vi "envoi mail valves expediées.vi"(4 "tab histo filtré\n par n° cmde":string[][](array[string]), 7 "DIVISION":enum16{"FLATPROP", "MEDIC"}(ring), 8 "error in (no error)":errorcluster caption="entrée d'erreur (pas d'erreur)", 10 "DATA cmde":T1, 11 "chaine valves":string="12-216C-04521 EQIFIL 417mA 14.4ohm\t112105740008030109\t18.04.2008 15:35\tMQI\t12345/06-03.03.03\t2\t30\r\n12-216C-04521 EQIFIL 417mA 14.4ohm\t112105740008030108\t18.04.2008 15:35\tMQI\t12345/06-03.03.03\t2\t30\r\n12-216C-04521 EQIFIL 417mA 14.4ohm\t112105740008030107\t18.04.2008 15:35\tMQI\t12345/06-03.03.03\t2\t30\r\n12-216C-04521 EQIFIL 417mA 14.4ohm\t112105740008030106\t18.04.2008 15:35\tMQI\t12345/06-03.03.03\t2\t30\r\n12-216C-04521 EQIFIL 417mA 14.4ohm\t112105740008030105\t18.04.2008 15:35\tMQI\t12345/06-03.03.03\t2\t30\r\n12-216C-04521 EQIFIL 417mA 14.4ohm\t112105740008030104\t18.04.2008 15:35\tMQI\t12345/06-03.03.03\t1\t30\r\n12-216C-04521 EQIFIL 417mA 14.4ohm\t112105740008030103\t18.04.2008 15:34\tMQI\t12345/06-03.03.03\t1\t30\r\n12-216C-04521 EQIFIL 417mA 14.4ohm\t112105740008030102\t18.04.2008 15:34\tMQI\t12345/06-03.03.03\t1\t30\r\n12-216C-04521 EQIFIL 417mA 14.4ohm\t112105740008030101\t18.04.2008 15:34\tMQI\t12345/06-03.03.03\t1\t30\r\n12-216C-04521 EQIFIL 417mA 14.4ohm\t112105740008030100\t18.04.2008 15:34\tMQI\t12345/06-03.03.03\t1\t30\r\n12-216C-04521 EQIFIL 417mA 14.4ohm\t112105740008020106\t18.04.2008 15:34\tMQI\t12345/06-03.03.03\t1\t30\r\n12-216C-04521 EQIFIL 417mA 14.4ohm\t112105740008020105\t18.04.2008 15:34\tMQI\t12345/06-03.03.03\t1\t30\r\n12-216C-04521 EQIFIL 417mA 14.4ohm\t112105740008020104\t18.04.2008 15:34\tMQI\t12345/06-03.03.03\t1\t30\r\n12-216C-04521 EQIFIL 417mA 14.4ohm\t112105740008020103\t18.04.2008 15:34\tMQI\t12345/06-03.03.03\t1\t30\r\n12-216C-04521 EQIFIL 417mA 14.4ohm\t112105740008020102\t18.04.2008 15:34\tMQI\t12345/06-03.03.03\t1\t30\r\n12-216C-04521 EQIFIL 417mA 14.4ohm\t112105740008020101\t18.04.2008 15:34\tMQI\t12345/06-03.03.03\t1\t30\r\n12-216C-04521 EQIFIL 417mA 14.4ohm\t112105740008020100\t18.04.2008 15:34\tMQI\t12345/06-03.03.03\t1\t30\r\n12-216C-04521 EQIFIL 417mA 14.4ohm\t112105740008010112\t18.04.2008 15:34\tMQI\t12345/06-03.03.03\t1\t30\r\n12-216C-04521 EQIFIL 417mA 14.4ohm\t112105740008010111\t18.04.2008 15:34\tMQI\t12345/06-03.03.03\t1\t30\r\n12-216C-04521 EQIFIL 417mA 14.4ohm\t112105740008010110\t18.04.2008 15:34\tMQI\t12345/06-03.03.03\t1\t30\r\n12-216C-04521 EQIFIL 417mA 14.4ohm\t112105740008010109\t18.04.2008 15:34\tMQI\t12345/06-03.03.03\t1\t30\r\n12-216C-04521 EQIFIL 417mA 14.4ohm\t112105740008010108\t18.04.2008 15:34\tMQI\t12345/06-03.03.03\t1\t30\r\n12-216C-04521 EQIFIL 417mA 14.4ohm\t112105740008010107\t18.04.2008 15:34\tMQI\t12345/06-03.03.03\t1\t30\r\n12-216C-04521 EQIFIL 417mA 14.4ohm\t112105740008010106\t18.04.2008 15:34\tMQI\t12345/06-03.03.03\t1\t30\r\n12-216C-04521 EQIFIL 417mA 14.4ohm\t112105740008010105\t18.04.2008 15:34\tMQI\t12345/06-03.03.03\t1\t30\r\n12-216C-04521 EQIFIL 417mA 14.4ohm\t112105740008010104\t18.04.2008 15:34\tMQI\t12345/06-03.03.03\t1\t30\r\n12-216C-04521 EQIFIL 417mA 14.4ohm\t112105740008010103\t18.04.2008 15:33\tMQI\t12345/06-03.03.03\t1\t30\r\n12-216C-04521 EQIFIL 417mA 14.4ohm\t112105740008010102\t18.04.2008 15:33\tMQI\t12345/06-03.03.03\t1\t30\r\n12-216C-04521 EQIFIL 417mA 14.4ohm\t112105740008010101\t18.04.2008 15:33\tMQI\t12345/06-03.03.03\t1\t30\r\n12-216C-04521 EQIFIL 417mA 14.4ohm\t112105740008010100\t18.04.2008 15:33\tMQI\t12345/06-03.03.03\t1\t30\r\n") -> (0 "error out":errorcluster caption="sortie d'erreur")   [LabVIEW 2020]
doc: "Envoi un mail avec la liste des valves emballées en pièce jointe si spécifié dans le fichier XML PP de la valve (FlatProp) ou correspondance produit code barre.txt (autres valves)"
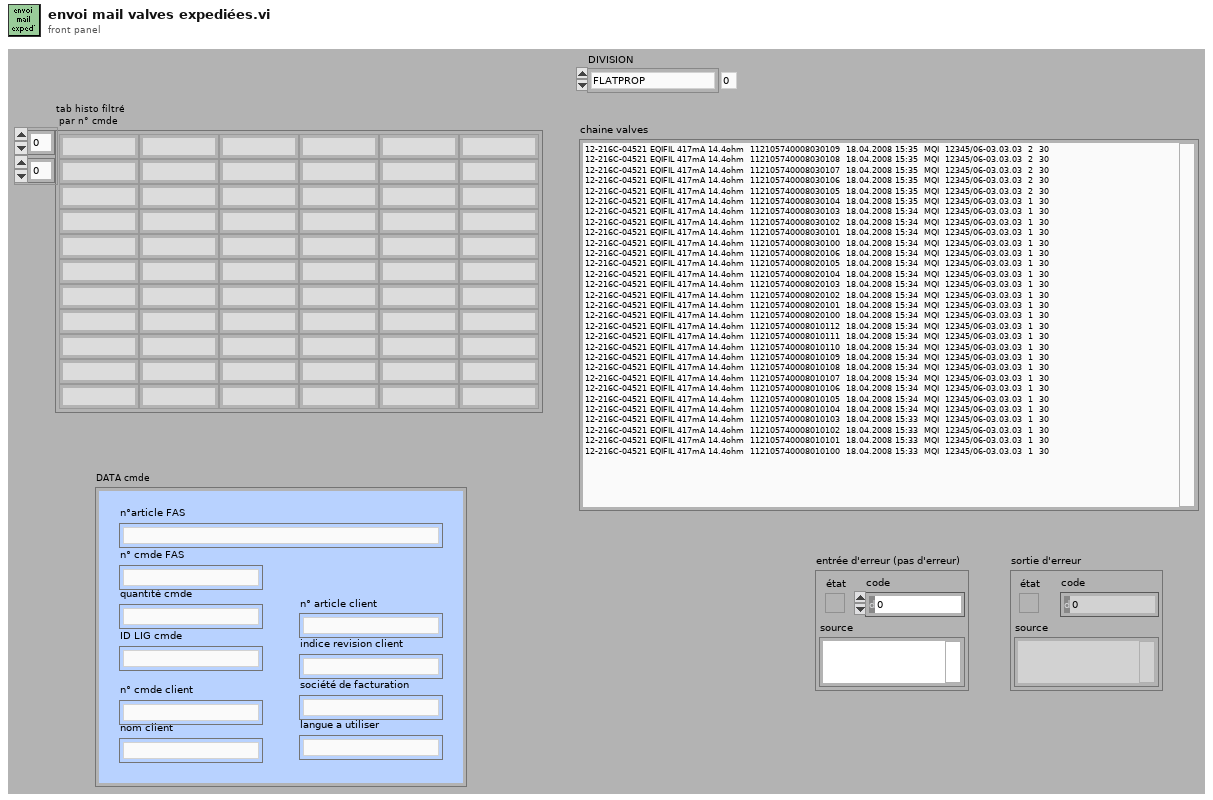
[diagram p1: front panel]
types:
  T1 = typedef "DATA commande.ctl" = cluster{"n°article FAS":string, "n° cmde FAS":string, "quantité cmde":string, "ID LIG cmde":string, "n° cmde client":string, "nom client":string, "n° article client":string, "indice revision client":string, "société de facturation":string, "langue a utiliser":string}
  T2 = enum16{"open", "replace", "create", "open or create", "replace or create", "replace or create with confirmation"}
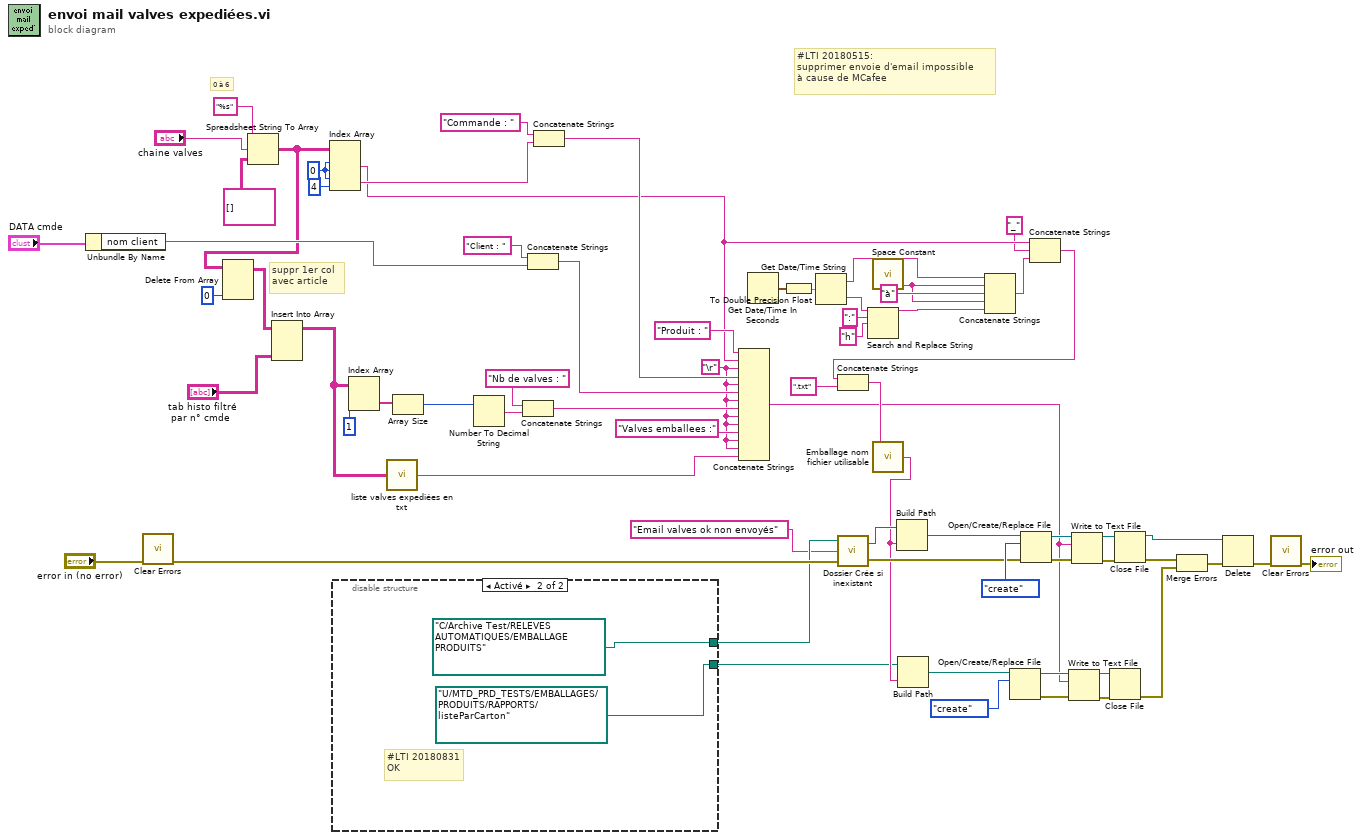
[diagram p0: block diagram]
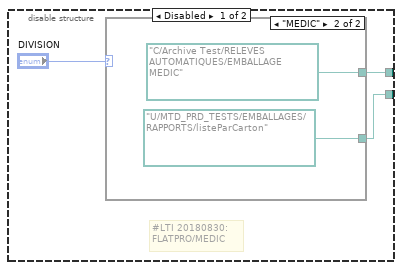
[diagram p2: hidden frame]
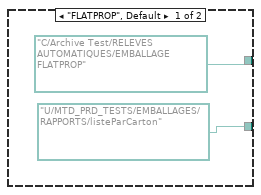
[diagram p3: hidden frame]
diagram:
  w52 = 0 ("indice désactivé (col)")
  w38 = "\r"
  # "#LTI 20180515:\nsupprimer envoie d'email impossible \nà cause de MCafee"
  # "suppr 1er col \navec article"
  # "0 à 6"
  n1 = Unbundle By Name("DATA cmde") -> ("nom client"=w65:string)
  n2 = call <vilib>:"Clear Errors.vi"("error in (no error)"="error in (no error)") -> ("error out"=w67:errorcluster)  [unwired: 5 in, 1 out]
  n3 = Spreadsheet String To Array(format string="%s" ("chaîne de format"), spreadsheet string="chaine valves", array type (2D Dbl)=string[][] [] ("type de tableau (2D de dbl)")) -> (array=w19:string[][])  [unwired: 1 in]
  n4 = Delete From Array(array=w19, index (col)=0 ("indice désactivé (col)")) -> (array with subset deleted=w17:string[][])  [unwired: 2 in, 1 out]
  n5 = Insert Into Array(array=w17, new element="tab histo filtré\n par n° cmde") -> (w14:string[][])  [unwired: 2 in]
  n6 = Index Array(array=w19, index (row) #1=w52, index (col) #1=w52, index (row) #2=w52, index (col) #2=4 ("indice désactivé (col)")) -> (element #1=w36:string, element #2=w50:string)
  n7 = disable-structure shown="Activé" {
    disable-tunnel: [w72 path "C:/Archive Test/RELEVES AUTOMATIQUES/EMBALLAGE PRODUITS" ("chemin local RELEVES AUTOM\\EMBALL_...")] -> w34
    disable-tunnel: [w70 path "U:/MTD_PRD_TESTS/EMBALLAGES/PRODUITS/RAPPORTS/listeParCarton" ("chemin local RELEVES AUTOM\\EMBALL_...")] -> w11
    frame Disabled {
      # "#LTI 20180830:\nFLATPRO/MEDIC"
      n8 = case shown="\"MEDIC\"" "DIVISION" {
        tunnel: [path "C:/Archive Test/RELEVES AUTOMATIQUES/EMBALLAGE FLATPROP" ("chemin local RELEVES AUTOM\\EMBALL_...") path "C:/Archive Test/RELEVES AUTOMATIQUES/EMBALLAGE MEDIC" ("chemin local RELEVES AUTOM\\EMBALL_...")] -> w72
        tunnel: [path "U:/MTD_PRD_TESTS/EMBALLAGES/RAPPORTS/listeParCarton" ("chemin local RELEVES AUTOM\\EMBALL_...") path "U:/MTD_PRD_TESTS/EMBALLAGES/RAPPORTS/listeParCarton" ("chemin local RELEVES AUTOM\\EMBALL_...")] -> w70
        frame "FLATPROP", Default {
        }
        frame "MEDIC" {
        }
      }
    }
    frame Enabled {
      # "#LTI 20180831\nOK"
    }
  }
  n9 = Index Array(array=w14, index (col)=1 ("indice désactivé (col)")) -> (element=w47:string[])  [unwired: 1 in]
  n10 = call "liste valves expediées en txt.vi"("Tab valves"=w14) -> ("liste valves"=w39:string)
  n11 = Array Size(array=w47) -> (size(s)=w16:i32)
  n12 = Number To Decimal String(number=w16) -> (decimal integer string=w45:string)  [unwired: 1 in]
  n13 = Concatenate Strings("Nb de valves : " ("expression régulière"), w45) -> (w62:string)
  n14 = Concatenate Strings("Client : " ("expression régulière"), w65) -> (w40:string)
  n15 = Concatenate Strings("Commande : " ("expression régulière"), w50) -> (w63:string)
  n16 = Concatenate Strings("Produit : " ("expression régulière"), w36, w38, w63, w38, w40, w38, w62, w38, w38, "Valves emballees :" ("chaîne"), w38, w38, w39) -> (w2:string)
  n17 = Get Date/Time In Seconds() -> (seconds since 1Jan1904=w28:timestamp)
  n18 = To Double Precision Float(number=w28) -> (double precision float=w29:dbl)
  n19 = Get Date/Time String(seconds (now)=w29) -> (date string=w22:string, time string=w25:string)  [unwired: 2 in]
  n20 = call "Dossier Crée si inexistant.vi"("error in"=w67, "nom sous dossier"="Email valves ok non envoyés", "chemin du dossier IN"=w34) -> ("error out"=w33:errorcluster, "chemin sous dossier OUT"=w31:path)
  n21 = Search and Replace String(input string=w25, search string=":" ("chaîne recherchée"), replace string="h" ("chaîne de remplacement (\"\")")) -> (result string=w23:string)  [unwired: 5 in, 3 out]
  n22 = call <vilib>:"Space Constant.vi"() -> ("String"=w21:string)
  n23 = Concatenate Strings(w22, w21, "à" ("chaîne"), w21, w23) -> (w20:string)
  n24 = Concatenate Strings(w36, "_", w20) -> (w35:string)
  n25 = Concatenate Strings(w35, ".txt" ("chaîne")) -> (w13:string)
  n26 = call "Emballage nom fichier utilisable.vi"("chaîne en entrée"=w13) -> ("chaîne résultante"=w12:string)
  n27 = Build Path(base path=w31, name or relative path=w12) -> (appended path=w32:path)
  n28 = Build Path(base path=w11, name or relative path=w12) -> (appended path=w5:path)
  n29 = Open/Create/Replace File(file path (use dialog)=w5, operation (0:open)=T2."create" ("opération (0 : open)")) -> (refnum out=w8:refnum<file>, error out=w6:errorcluster)  [unwired: 4 in, 1 out]
  n30 = Open/Create/Replace File(file path (use dialog)=w32, error in=w33, operation (0:open)=T2."create" ("opération (0 : open)")) -> (refnum out=w59:refnum<file>, error out=w61:errorcluster)  [unwired: 3 in, 1 out]
  n31 = Write to Text File(file (use dialog)=w8, text=w2, error in=w6) -> (refnum out=w10:refnum<file>, error out=w9:errorcluster)  [unwired: 1 in, 1 out]
  n32 = Write to Text File(file (use dialog)=w59, text=w2, error in=w61) -> (refnum out=w57:refnum<file>, error out=w58:errorcluster)  [unwired: 1 in, 1 out]
  n33 = Close File(refnum=w10, error in=w9) -> (error out=w3:errorcluster)  [unwired: 1 out]
  n34 = Close File(refnum=w57, error in=w58) -> (path=w37:path, error out=w56:errorcluster)
  n35 = Merge Errors(w56, w3) -> (w4:errorcluster)
  n36 = Delete(path (use dialog)=w37, error in=w4) -> (error out=w42:errorcluster)  [unwired: 3 in, 2 out]
  n37 = call <vilib>:"Clear Errors.vi"("error in (no error)"=w42) -> ("error out"=→"error out":errorcluster)  [unwired: 5 in, 1 out]
